vi "ex_cleanUpComment.vi"(1 "comment":string) -> (0 "output":string)   [LabVIEW 2020]
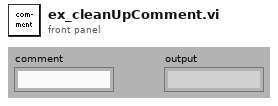
[diagram p1: front panel]
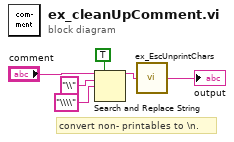
[diagram p0: block diagram]
diagram:
  # "convert non- printables to \\n."
  n1 = Search and Replace String(replace all?=TRUE, input string="comment", search string="\\" ("regular expression"), replace string="\\\\") -> (result string=w3:string)  [unwired: 1 in, 6 out]
  n2 = call <vilib>:"ex_EscUnprintChars.vi"("input"=w3) -> ("output"=→"output":string)
